vi "EM Machine Example.vi"(8 "error in":errorcluster) -> (0 "error out":errorcluster)   [LabVIEW 2013, in "daqio minimal.lvlib"]
doc: "This interactive example demonstrates how a device or machine could continuously publish data to daq.io. When correct user credentials are given, it will log on to daq.io, autocreate all device settings if required and will update time series values continuously. When changing the tag values (or Tags), these will be updated as well. When firing an Event, it will become visible on the daq.io events page. \n\nRefer to the Embedded example for an example that can easily be run on a RIO platform continuously."
uses:
  daqio minimal.lvlib
  _typedefs/update-button.ctl
  _typedefs/trigger-button.ctl
  _typedefs/exmpl_overlay_mask.ctl
  _typedefs/dashboard-button.ctl
  _typedefs/exmpl-states.ctl
  _typedefs/daqio-Credentials.ctl
  _typedefs/daqio-Type.ctl
  <vilib>/httpClient/ClientHandle.ctl
  _subs/daqio_Write_Multiple_single_Timestamp.vi
  <vilib>/httpClient/LabVIEWHTTPClient.lvlib
panel:
  out "overlay mask":T1
  in  "Create Dashboard":T2
  out "Log":string[](array[string])
  in  "Stop":bool
  in  "Fire Event":T3
  in  "Select Event":u16(ring) items=["Safety Hood Status", "Manual Operation", "Shutting Down"]
  out "Time Stamp sent":timestamp
  in  "Event Data":string
  in  "Update Tags":T4
  out "connected to daq.io":bool
  out "Speed (RPM)":dbl(knob) scale=0.0..2000.0
  out "Temperature Data":dbl(graph)
  out "RAM":dbl(slide) scale=0.0..100.0
  out "CPU":dbl(slide) scale=0.0..100.0
  in  "Setpoint\n(set manually)":dbl(knob) scale=0.0..100.0
  in  "Value 3":string="1234-abc"
  in  "Value 2":string="XYZ 3000 Plus"
  in  "Tag 3":string="Serial Number"
  in  "Tag 2":string="Type"
  in  "Value 1":string="47.615459, -122.323804"
  in  "Tag 1":string="Location"
  out "Device Key":string
  out "Device Type Key":string
  in  "Log On":bool
  in  "User Name":string
  in  "Password":string
  out "Dashboard URL - copy and open in your web browser":string
  # "This Machine"
  # "(autogenerated in this example)"
  # "Device Tags"
  # "Use device tags to describe \nspecific parameters for each\ndevice. These can include the \nlocation, the serial number or\nother machine or location-\nspecific information. These\nfields are fully user-defined."
  # "Device Events"
  # "Use device events to signal\nany local event to daq.io. These\ncould include mechanical events\n(e.g. \"safety latch released\") or \nany change on the device that\nneeds to be tracked."
  # "Device Live Data Channels"
  # "Use device channels to transfer\ntime series data. All channels \nof the device will be visible in \nthe online data viewer. You \ncan build your own dashboard \nin the webbrowser and link it\nto exisiting channels. Clicking\n\"Create Dashboard\" will\ngenerate a dashboard \nfor this example."
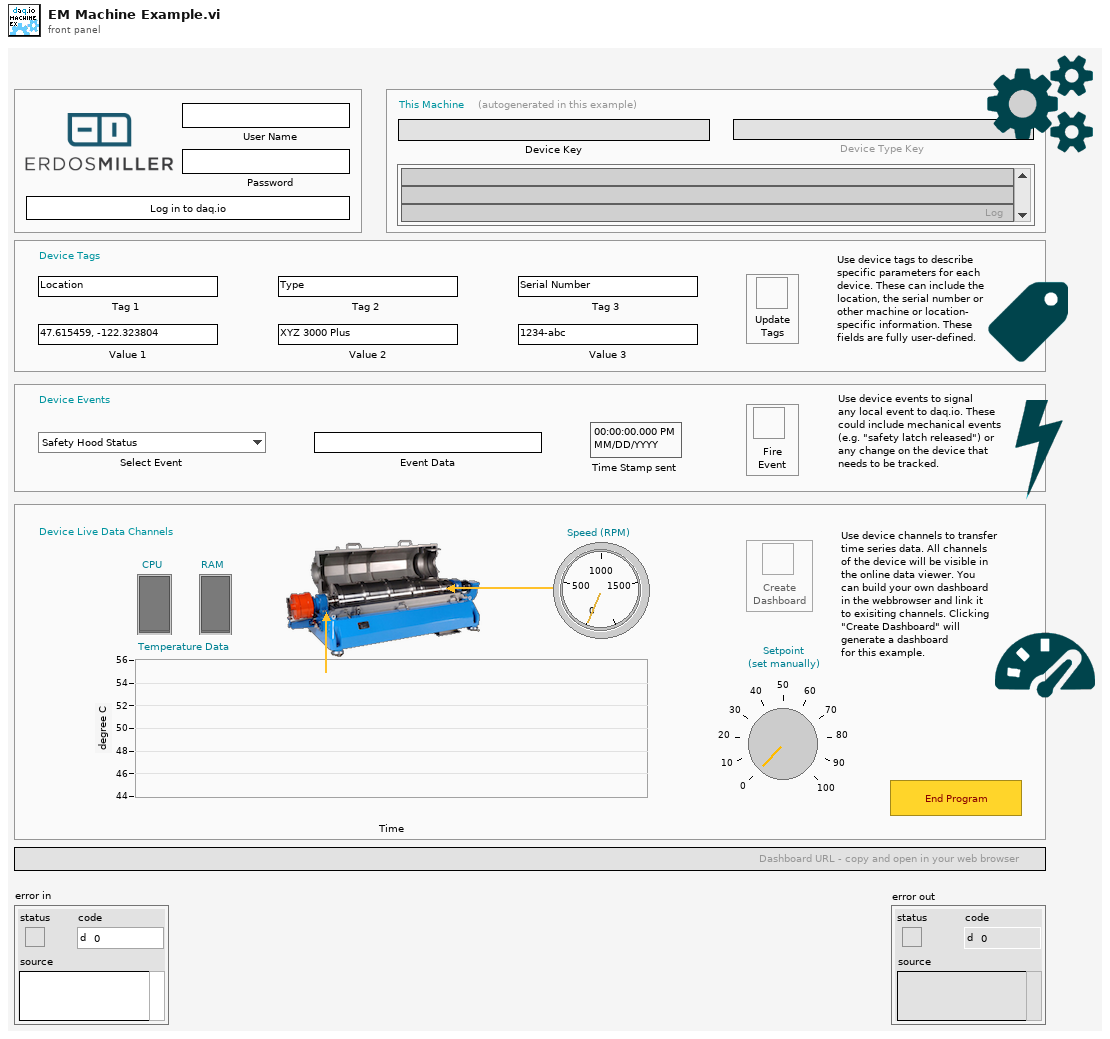
[diagram p1: front panel]
types:
  T1 = typedef "daqio minimal.lvlib/exmpl_overlay_mask.ctl" = bool
  T2 = typedef "daqio minimal.lvlib/dashboard-button.ctl" = bool
  T3 = typedef "daqio minimal.lvlib/trigger-button.ctl" = bool
  T4 = typedef "daqio minimal.lvlib/update-button.ctl" = bool
  T5 = typedef "daqio minimal.lvlib/exmpl-states.ctl" = enum16{"idle", "time series", "fire events", "update tags", "end program", "create dashboard"}
  T6 = typedef "daqio minimal.lvlib/daqio-Credentials.ctl" = cluster{"User Name":string, "Password":string}
  T7 = typedef "daqio minimal.lvlib/daqio-Type.ctl" = cluster{"daq.io ref":T8, "daq.io API Base":string, "Device Type Key":string, "Device Key":string, "Account ID":string, "online":bool}
  T8 = typedef "LabVIEWHTTPClient.lvlib/ClientHandle.ctl" = refnum<k1>
  T9 = enum8{"Enabled", "Disabled", "Disabled and Grayed Out"}
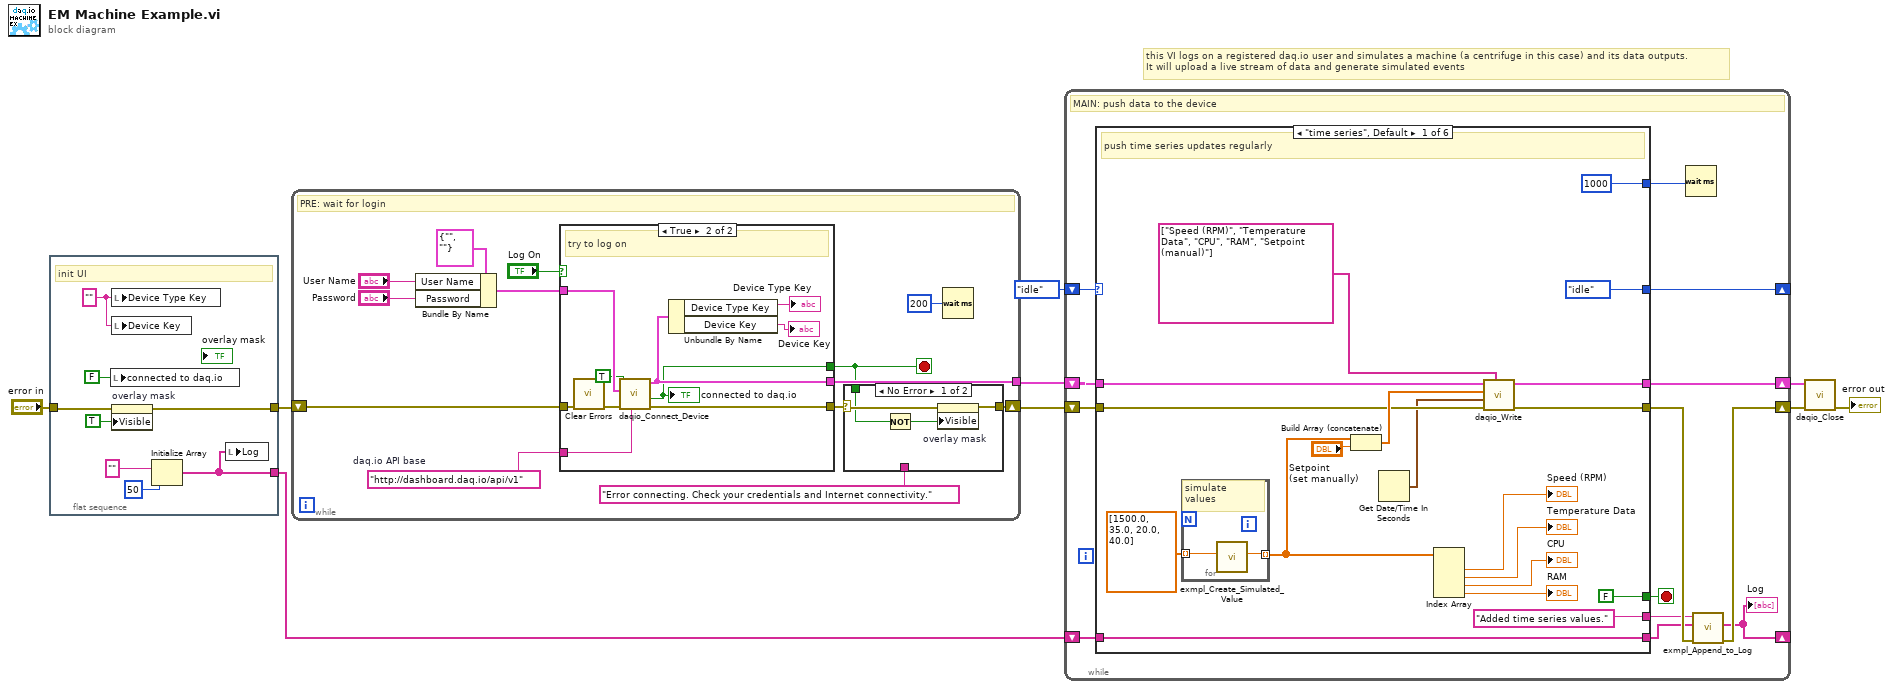
[diagram p0: block diagram]
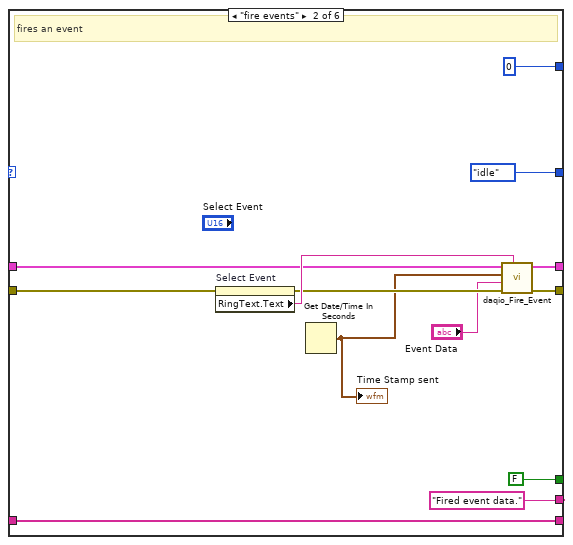
[diagram p2: hidden frame]
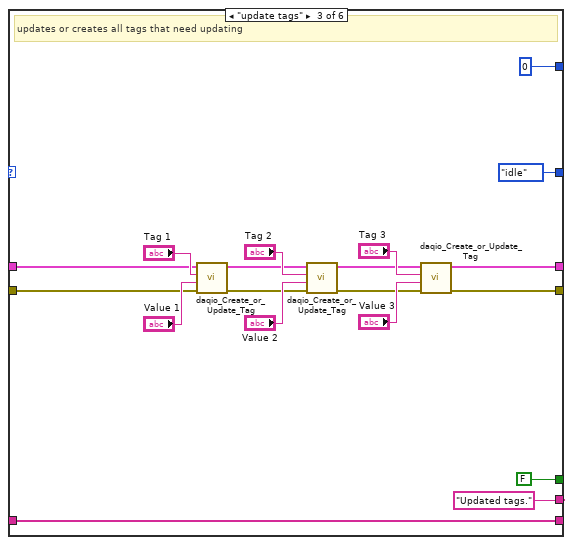
[diagram p3: hidden frame]
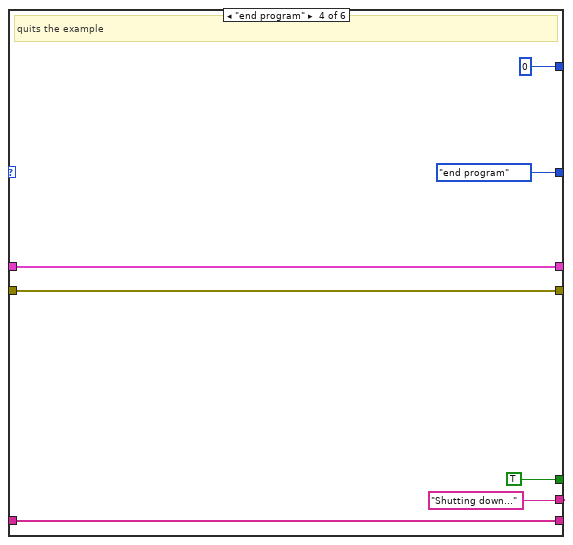
[diagram p4: hidden frame]
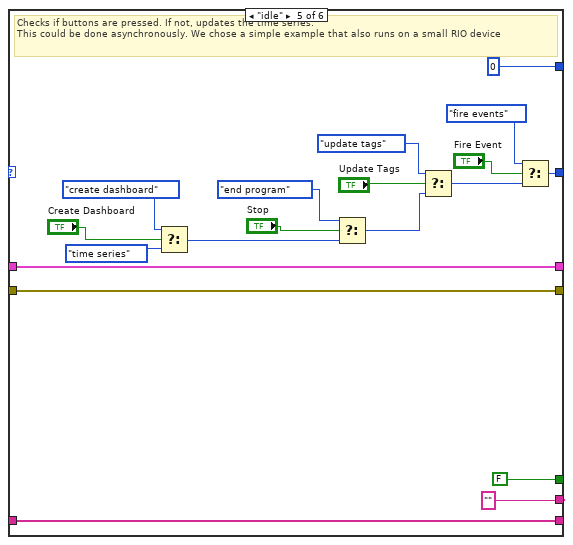
[diagram p5: hidden frame]
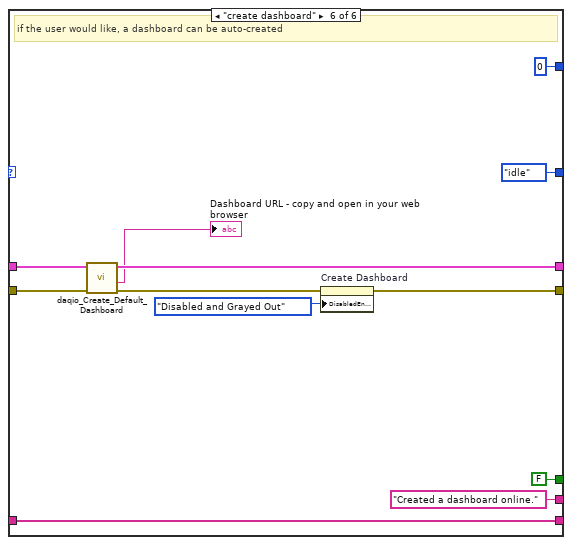
[diagram p6: hidden frame]
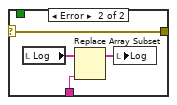
[diagram p7: hidden frame]
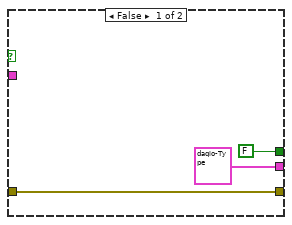
[diagram p8: hidden frame]
diagram:
  # "this VI logs on a registered daq.io user and simulates a machine (a centrifuge in this case) and its data outputs. \nIt will upload a live stream of data and generate simulated events"
  n1 = flat-sequence {
    tunnel: [w14] -> w6
    tunnel: "error in" -> [w15]
    tunnel: [w10] -> w1
    frame #0 {
      w17 = "" ("log")
      # "init UI"
      n2 = local write "connected to daq.io"(FALSE ("connected to daq.io")) -> ()
      n3 = local write "Device Type Key"(w17) -> ()
      n4 = local write "Device Key"(w17) -> ()
      n5 = property on="overlay mask" class="Bool (strict)"(error in=w15, "Visible"=TRUE) -> (error out=w14:errorcluster)  [unwired: 1 in, 1 out]
      n6 = Initialize Array("" ("log"), 50 ("dimension size")) -> (w10:string[])
      n7 = local write "Log"(w10) -> ()
    }
  }
  n8 = while {
    shift-right: [w20] -> w4
    shift-left: w6 -> [w18]
    tunnel: [w25] -> w5
    stop <- w19 stop-if-true
    w23 = "http://dashboard.daq.io/api/v1"  # daq.io API base
    # "PRE: wait for login"
    n9 = Bundle By Name(cluster=T6 {"User Name"="", "Password"=""} ("daq.io Credentials"), "User Name"="User Name", "Password"="Password") -> (w24:T6)
    n10 = case shown="True" "Log On" {
      tunnel: [T7 {"daq.io ref"=refnum, "daq.io API Base"="http://dashboard.daq.io/api/v1", "Device Type Key"="", "Device Key"="", "Account ID"="", "online"=FALSE} ("daq.io type out") w47] -> w25
      tunnel: [w39 w51] -> w21
      tunnel: w18 -> [w39 w50]
      tunnel: w23 -> [_ w49]
      tunnel: w24 -> [_ w48]
      tunnel: [FALSE ("connected successfully?") w44] -> w19
      frame False {
      }
      frame True {
        # "try to log on"
        n11 = call <vilib>:"Clear Errors.vi"("error in (no error)"=w50) -> ("error out"=w43:errorcluster)  [unwired: 6 in]
        n12 = call "daqio_Connect_Device.vi"("daq.io API base"=w49, "error in (no error)"=w43, "Credentials"=w48, "Use System Status Event?"=TRUE) -> ("error out"=w51:errorcluster, "connected successfully?"=w44:bool, "daq.io type out"=w47:T7)  [unwired: 4 in, 1 out]
        "connected to daq.io" <- w44
        n13 = Unbundle By Name(w47) -> ("Device Type Key"=→"Device Type Key":string, "Device Key"=→"Device Key":string)
      }
    }
    n14 = case shown="No Error" w21 {
      selector: w21 -> [w33 w35]
      tunnel: "Error connecting. Check your credentials and Internet connectivity." ("new element/subarray") -> [_ w36]
      tunnel: [w34 w35] -> w20
      tunnel: w19 -> [w32 _]
      frame No Error {
        n15 = Not(x=w32) -> (.not. x?=w31:bool)
        n16 = property on="overlay mask" class="Bool (strict)"(error in=w33, "Visible"=w31) -> (error out=w34:errorcluster)  [unwired: 1 in, 1 out]
      }
      frame Error {
        n17 = local read "Log"() -> (w38:string[])
        n18 = Replace Array Subset(array=w38, new element=w36) -> (w37:string[])  [unwired: 1 in]
        n19 = local write "Log"(w37) -> ()
      }
    }
    n20 = Wait (ms)(milliseconds to wait=u32 200) -> ()  [unwired: 1 out]
  }
  n21 = while {
    shift-right: [w55] -> w9
    shift-left: w4 -> [w63]
    shift-right: [w62] -> w3
    shift-left: w5 -> [w64]
    shift-right: [w60] -> _
    shift-left: exmpl-states."idle" -> [w61]
    shift-right: [w52] -> _
    shift-left: w1 -> [w57]
    stop <- w59 stop-if-true
    # "MAIN: push data to the device"
    n22 = case shown="\"time series\", Default" w61 {
      tunnel: w64 -> [w71 w95 w107 w122 w139 w150]
      tunnel: w63 -> [w68 w94 w106 w121 w138 w149]
      tunnel: [w65 w92 w104 w122 w139 w148] -> w62
      tunnel: [w66 w93 w105 w121 w138 w144] -> w56
      tunnel: [exmpl-states."idle" exmpl-states."idle" exmpl-states."idle" exmpl-states."end program" w140 exmpl-states."idle"] -> w60
      tunnel: [FALSE FALSE FALSE TRUE FALSE FALSE] -> w59
      tunnel: [u32 1000 ("milliseconds to wait") u32 0 ("milliseconds to wait") u32 0 ("milliseconds to wait") u32 0 ("milliseconds to wait") u32 0 ("milliseconds to wait") u32 0 ("milliseconds to wait")] -> w58
      tunnel: ["Added time series values." ("log") "Fired event data." ("log") "Updated tags." ("log") "Shutting down..." ("log") "" "Created a dashboard online." ("log")] -> w54
      tunnel: w57 -> [w73 w87 w99 w118 w129 w155]
      tunnel: [w73 w87 w99 w118 w129 w155] -> w53
      frame "time series", Default {
        # "push time series updates regularly"
        n23 = for {
          tunnel: [w85] -> w82 mode=indexing
          tunnel: dbl[] [1500.0, 35.0, 20.0, 40.0] -> [w84] mode=indexing
          # "simulate\nvalues"
          n24 = call "exmpl_Create_Simulated_Value.vi"("offset"=w84) -> ("Numeric"=w85:dbl)  [unwired: 9 in, 1 out]
        }
        n25 = Build Array (concatenate)(w82, "Setpoint\n(set manually)") -> (w69:dbl[])
        n26 = Get Date/Time In Seconds() -> (seconds since 1Jan1904=w67:timestamp)
        n27 = Index Array(array=w82) -> (element #1=→"Speed (RPM)":dbl, element #2=→"Temperature Data":dbl, element #3=→"CPU":dbl, element #4=→"RAM":dbl)  [unwired: 4 in]
        n28 = call-poly "daqio_Write.vi"("daq.io Device Channels"=string[] ["Speed (RPM)", "Temperature Data", "CPU", "RAM", "Setpoint (manual)"], "error in (no error)"=w68, "Timestamp"=w67, "Values"=w69, "daq.io type in"=w71) -> ("error out"=w66:errorcluster, "daq.io type out"=w65:T7)  [unwired: 5 in]
      }
      frame "fire events" {
        # "fires an event"
        n29 = property on="Select Event" class="Ring (strict)"(error in=w94) -> (error out=w97:errorcluster, "RingText.Text"=w98:string)  [unwired: 1 in, 1 out]
        n30 = Get Date/Time In Seconds() -> (seconds since 1Jan1904=w86:timestamp)
        "Time Stamp sent" <- w86
        n31 = call "daqio_Fire_Event.vi"("Event Key"=w98, "error in (no error)"=w97, "Event Value"="Event Data", "Event Date and Time"=w86, "daq.io type in"=w95) -> ("error out"=w93:errorcluster, "daq.io type out"=w92:T7)  [unwired: 5 in]
      }
      frame "update tags" {
        # "updates or creates all tags that need updating"
        n32 = call "daqio_Create_or_Update_Tag.vi"("error in (no error)"=w106, "Tag Value"="Value 1", "Tag Key"="Tag 1", "daq.io type in"=w107) -> ("error out"=w111:errorcluster, "daq.io type out"=w108:T7)  [unwired: 5 in, 1 out]
        n33 = call "daqio_Create_or_Update_Tag.vi"("error in (no error)"=w111, "Tag Value"="Value 2", "Tag Key"="Tag 2", "daq.io type in"=w108) -> ("error out"=w110:errorcluster, "daq.io type out"=w109:T7)  [unwired: 5 in, 1 out]
        n34 = call "daqio_Create_or_Update_Tag.vi"("error in (no error)"=w110, "Tag Value"="Value 3", "Tag Key"="Tag 3", "daq.io type in"=w109) -> ("error out"=w105:errorcluster, "daq.io type out"=w104:T7)  [unwired: 5 in, 1 out]
      }
      frame "end program" {
        # "quits the example"
      }
      frame "idle" {
        # "Checks if buttons are pressed. If not, updates the time series. \nThis could be done asynchronously. We chose a simple example that also runs on a small RIO device"
        n35 = Select(t=exmpl-states."create dashboard", s="Create Dashboard", f=exmpl-states."time series") -> (s? t:f=w125:T5)
        n36 = Select(t=exmpl-states."end program", s="Stop", f=w125) -> (s? t:f=w132:T5)
        n37 = Select(t=exmpl-states."update tags", s="Update Tags", f=w132) -> (s? t:f=w141:T5)
        n38 = Select(t=exmpl-states."fire events", s="Fire Event", f=w141) -> (s? t:f=w140:T5)
      }
      frame "create dashboard" {
        # "if the user would like, a dashboard can be auto-created"
        n39 = call "daqio_Create_Default_Dashboard.vi"("error in (no error)"=w149, "daq.io type in"=w150) -> ("error out"=w145:errorcluster, "Dashboard URL"=→"Dashboard URL - copy and open in your web browser":string, "daq.io type out"=w148:T7)  [unwired: 6 in, 1 out]
        n40 = property on="Create Dashboard" class="Bool"(error in=w145, "DisabledEnum"=T9."Disabled and Grayed Out" ("Disabled")) -> (error out=w144:errorcluster)  [unwired: 1 in, 1 out]
      }
    }
    n41 = Wait (ms)(milliseconds to wait=w58) -> ()  [unwired: 1 out]
    n42 = call "exmpl_Append_to_Log.vi"("error in (no error)"=w56, "Log Array in"=w53, "Log Message"=w54) -> ("error out"=w55:errorcluster, "Log Array out"=w52:string[])  [unwired: 7 in]
    "Log" <- w52
  }
  n43 = call "daqio_Close.vi"("error in (no error)"=w9, "daq.io type"=w3) -> ("error out"=→"error out":errorcluster)  [unwired: 9 in]
